vi "Configure Burst.vi"(4 "Burst Period (1 s)":dbl=1.0 min=0.002 max=1000000.0 format="%.6f", 6 "Burst Count (1)":i32=1, 7 "Burst Mode (0: Triggered)":u16(ring) items=["Triggered", "Gated"], 8 "error in (no error)":errorcluster, 9 "Burst Phase (0 deg)":i32 min=-360 max=360, 10 "Enable Burst (T: Enable)":bool=TRUE, 11 "VISA resource name":refnum<visa-resource-name>) -> (0 "error out":errorcluster, 3 "VISA resource name out":refnum<visa-resource-name>)   [LabVIEW 2018, in "AWG.lvlib" / "Agilent 33XXX Series.lvlib"]
doc: "Allows and configures burst. Configures the function generator to output a waveform with specified number of cycles, called burst. The carrier waveform shape and parameters are set by Configure Standard Waveform.\nUse negative burst count to enable infinite pulse count.\n\nNote:\n(1) Before using this mode, all other modes must be turned off.\n(2) This VI is valid in 33210, 33220, and 33250."
uses:
  Agilent 33XXX Series.lvlib
panel:
  # "Triggered BM Settings"
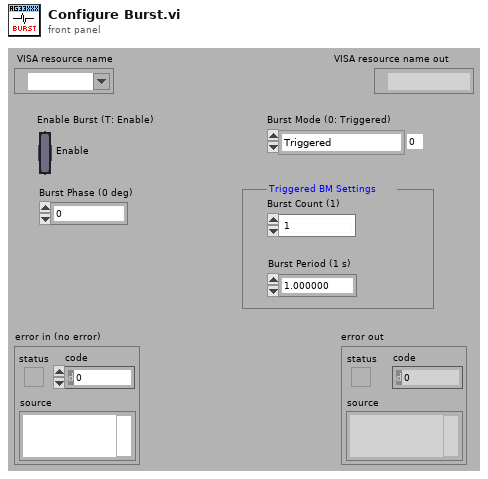
[diagram p1: front panel]
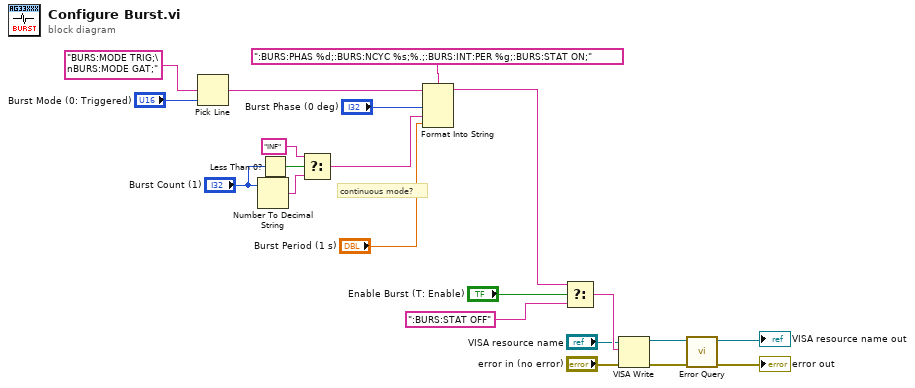
[diagram p0: block diagram]
diagram:
  # "continuous mode?"
  n1 = Pick Line(multi-line string="BURS:MODE TRIG;\nBURS:MODE GAT;" ("f"), line index="Burst Mode (0: Triggered)") -> (output string=w11:string)  [unwired: 1 in]
  n2 = Number To Decimal String(number="Burst Count (1)") -> (decimal integer string=w3:string)  [unwired: 1 in]
  n3 = Less Than 0?(x="Burst Count (1)") -> (x < 0?=w5:bool)
  n4 = Select(t="INF", s=w5, f=w3) -> (s? t:f=w1:string)
  n5 = Format Into String(format string=":BURS:PHAS %d;:BURS:NCYC %s;%.;:BURS:INT:PER %g;:BURS:STAT ON;", initial string=w11, "Burst Phase (0 deg)", w1, "Burst Period (1 s)") -> (resulting string=w10:string)  [unwired: 1 in, 1 out]
  n6 = Select(t=w10, s="Enable Burst (T: Enable)", f=":BURS:STAT OFF") -> (s? t:f=w9:string)
  n7 = VISA Write(VISA resource name="VISA resource name", write buffer=w9, error in (no error)="error in (no error)") -> (VISA resource name out=w21:refnum<visa-resource-name>, error out=w20:errorcluster)  [unwired: 1 out]
  n8 = call "Error Query.vi"("error in (no error)"=w20, "VISA resource name"=w21) -> ("error out"=→"error out":errorcluster, "VISA resource name out"=→"VISA resource name out":refnum<visa-resource-name>)  [unwired: 6 in, 2 out]
